vi "CheckTemperature.vi"(8 "error in (no error)":errorcluster, 11 "temperature in":i32) -> (0 "error out":errorcluster, 2 "TemperatureReached":bool)   [LabVIEW 2013]
uses:
  Utilities/controls/ctlSeqFNs_Andor_temp.ctl
  lib/atmcd32d.llb/Error Code Enum typedef.ctl
  Variables/GlobalGetTemperatureCamera.vi
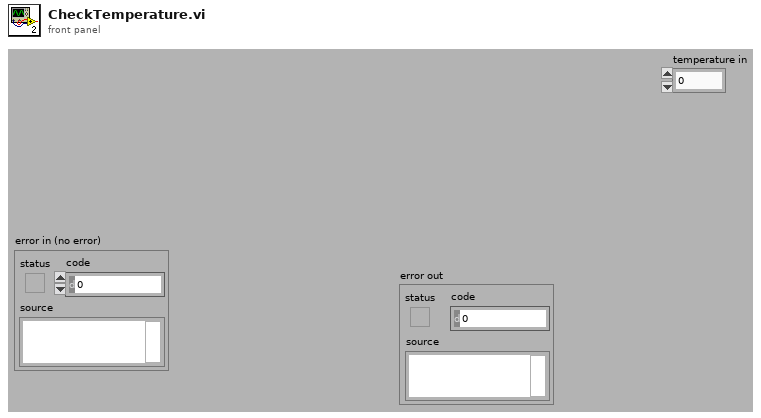
[diagram p1: front panel]
types:
  T1 = typedef "ctlSeqFNs_Andor_temp.ctl" = enum16{"Temperature  FALSE", "Temperature OK"}
  T2 = typedef "Error Code Enum typedef.ctl" = enum32{"N/A (0)", "DRV_ERROR_CODES", "DRV_SUCCESS", "DRV_VXDNOTINSTALLED", "DRV_ERROR_SCAN", "DRV_ERROR_CHECK_SUM", "DRV_ERROR_FILELOAD", "DRV_UNKNOWN_FUNC", "DRV_ERROR_VXD_INIT", "DRV_ERROR_ADDRESS", "DRV_ERROR_PAGELOCK", "DRV_ERROR_PAGEUNLOCK", "DRV_ERROR_BOARDTEST", "DRV_ERROR_ACK", "DRV_ERROR_UP_FIFO", "DRV_ERROR_PATTERN", "N/A (16)", "DRV_ACQUISITION_ERRORS", "DRV_ACQ_BUFFER", "DRV_ACQ_DOWNFIFO_FULL", "DRV_PROC_UNKONWN_INSTRUCTION", "DRV_ILLEGAL_OP_CODE", "DRV_KINETIC_TIME_NOT_MET", "DRV_ACCUM_TIME_NOT_MET", "DRV_NO_NEW_DATA", "N/A (25)", "DRV_SPOOLERROR", "N/A (27)", "N/A (28)", "N/A (29)", "N/A (30)", "N/A (31)", "N/A (32)", "DRV_TEMPERATURE_CODES", "DRV_TEMPERATURE_OFF", "DRV_TEMPERATURE_NOT_STABILIZED", "DRV_TEMPERATURE_STABILIZED", "DRV_TEMPERATURE_NOT_REACHED", "DRV_TEMPERATURE_OUT_RANGE", "DRV_TEMPERATURE_NOT_SUPPORTED", "DRV_TEMPERATURE_DRIFT", "N/A (41)", "N/A (42)", "N/A (43)", "N/A (44)", "N/A (45)", "N/A (46)", "N/A (47)", "N/A (48)", "DRV_GENERAL_ERRORS", "DRV_INVALID_AUX", "DRV_COF_NOTLOADED", "DRV_FPGAPROG", "DRV_FLEXERROR", "DRV_GPIBERROR", "N/A (55)", "N/A (56)", "N/A (57)", "N/A (58)", "N/A (59)", "N/A (60)", "N/A (61)", "N/A (62)", "N/A (63)", "DRV_DATATYPE", "DRV_DRIVER_ERRORS", "DRV_P1INVALID", "DRV_P2INVALID", "DRV_P3INVALID", "DRV_P4INVALID", "DRV_INIERROR", "DRV_COFERROR", "DRV_ACQUIRING", "DRV_IDLE", "DRV_TEMPCYCLE", "DRV_NOT_INITIALIZED", "DRV_P5INVALID", "DRV_P6INVALID", "DRV_INVALID_MODE", "DRV_INVALID_FILTER", "DRV_I2CERRORS", "DRV_I2CDEVNOTFOUND", "DRV_I2CTIMEOUT", "DRV_P7INVALID", "N/A (84)", "N/A (85)", "N/A (86)", "N/A (87)", "N/A (88)", "N/A (89)", "DRV_IOCERROR", "DRV_VRMVERSIONERROR"}
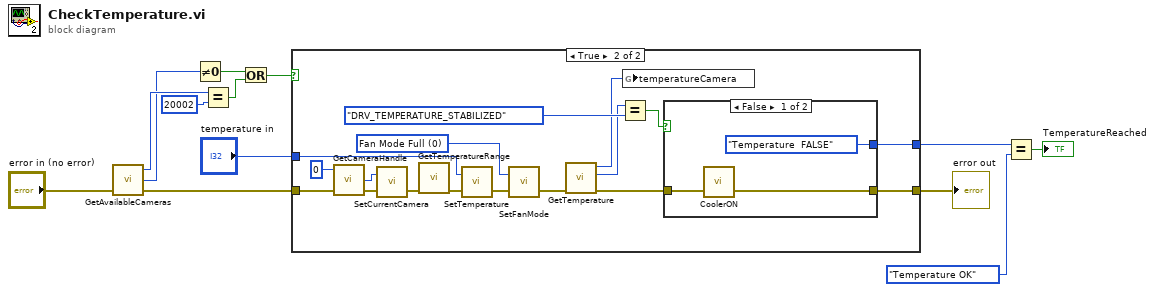
[diagram p0: block diagram]
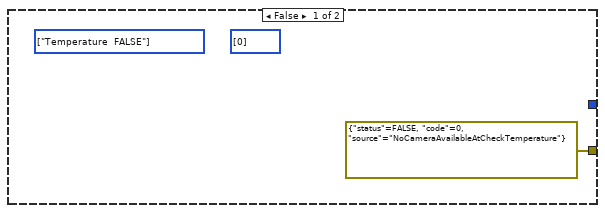
[diagram p2: hidden frame]
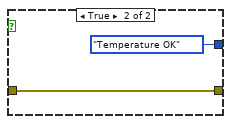
[diagram p3: hidden frame]
diagram:
  n1 = call "GetAvailableCameras.vi"("error in (no error)"="error in (no error)") -> ("error out"=w7:errorcluster, "totalCameras"=w6:i32, "DLL error code"=w13:u32)  [unwired: 2 in]
  n2 = Not Equal To 0?(x=w6) -> (x != 0?=w3:bool)
  n3 = Equal?(x=w13, y=u32 20002) -> (x = y?=w11:bool)
  n4 = Or(x=w3, y=w11) -> (x .or. y?=w9:bool)
  n5 = case shown="True" w9 {
    tunnel: [errorcluster {"status"=FALSE, "code"=0, "source"="NoCameraAvailableAtCheckTemperature"} ("error out") w31] -> w8
    tunnel: w7 -> [_ w30]
    tunnel: "temperature in" -> [_ w29]
    tunnel: [_ w16] -> w2
    frame False {
      (unwired) i32[] [0]
      (unwired) T1[] [enum."Temperature  FALSE"] items=["Temperature  FALSE", "Temperature OK"]
    }
    frame True {
      w26 = u16 0 items=["Fan Mode Full", "Fan Mode Half", "Fan Mode Low"] ("Ring")
      n6 = call "GetCameraHandle.vi"("error in (no error)"=w30, "cameraIndex"=0) -> ("error out"=w24:errorcluster, "cameraHandle"=w19:i32)  [unwired: 1 in, 1 out]
      n7 = call "SetCurrentCamera.vi"("error in (no error)"=w24, "cameraHandle"=w19) -> ("error out"=w18:errorcluster)  [unwired: 1 out]
      n8 = call "GetTemperatureRange.vi"("error in (no error)"=w18) -> ("error out"=w28:errorcluster)  [unwired: 3 in, 3 out]
      n9 = call "SetTemperature.vi"("error in (no error)"=w28, "temperature"=w29) -> ("error out"=w27:errorcluster)  [unwired: 1 out]
      n10 = call "SetFanMode.vi"("error in (no error)"=w27, "mode"=w26) -> ("error out"=w25:errorcluster)  [unwired: 1 out]
      n11 = call "GetTemperature.vi"("error in (no error)"=w25) -> ("error out"=w21:errorcluster, "status"=w22:T2, "temperature"=w17:i32)  [unwired: 3 in, 1 out]
      n12 = Equal?(x=w22, y=Error_Code_Enum_typedef."DRV_TEMPERATURE_STABILIZED" ("status")) -> (x = y?=w20:bool)
      n13 = global write "GlobalGetTemperatureCamera.vi" "temperatureCamera"(w17) -> ()
      n14 = case shown="False" w20 {
        tunnel: [ctlSeqFNs_Andor_temp."Temperature  FALSE" ("STATE") ctlSeqFNs_Andor_temp."Temperature OK" ("STATE")] -> w16
        tunnel: w21 -> [w33 w35]
        tunnel: [w32 w35] -> w31
        frame False {
          n15 = call "CoolerON.vi"("error in (no error)"=w33) -> ("error out"=w32:errorcluster)  [unwired: 1 in, 1 out]
        }
        frame True {
        }
      }
    }
  }
  "error out" <- w8
  n16 = Equal?(x=w2, y=ctlSeqFNs_Andor_temp."Temperature OK" ("STATE")) -> (x = y?=→"TemperatureReached":bool)
